vi "Get project path.vi"(1 "Project Name":string) -> (0 "Project path":path)   [LabVIEW 2012]
uses:
  <userlib>/_OpenG.lib/file/file.llb/Strip Path - Traditional__ogtk.vi
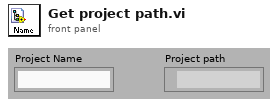
[diagram p1: front panel]
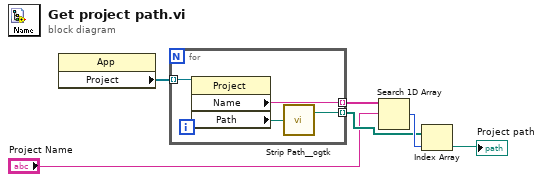
[diagram p0: block diagram]
diagram:
  n1 = property class="App"() -> ("Project"=w1:refnum<vi>[])  [unwired: 2 in, 2 out]
  n2 = for {
    tunnel: w1 -> [w10] mode=indexing
    tunnel: [w8] -> w4 mode=indexing
    tunnel: [w7] -> w2 mode=indexing
    n3 = property class="Project"(reference=w10) -> ("Name"=w7:string, "Path"=w9:path)  [unwired: 1 in, 2 out]
    n4 = call-poly <userlib>:"Strip Path__ogtk.vi"("path"=w9) -> ("stripped path"=w8:path)  [unwired: 1 out]
  }
  n5 = Search 1D Array(1D array=w2, element="Project Name") -> (index of element=w5:i32)  [unwired: 1 out]
  n6 = Index Array(array=w4, index=w5) -> (element=→"Project path":path)
